vi "Get Time.vi"() -> (0 "time (ns)":u64)   [LabVIEW 2015, in "FPGA Timekeeper.lvlib"]
doc: "Returns the current time of the FPGA Timekeeper."
uses:
  FPGA Timekeeper.lvlib
  private/time (g).vi
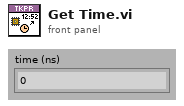
[diagram p1: front panel]
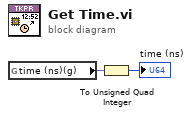
[diagram p0: block diagram]
diagram:
  n1 = global read "time (g).vi" "time (ns)(g)"() -> (w2:fxp<+,64,64>)
  n2 = To Unsigned Quad Integer(1:w2) -> (0:→"time (ns)":u64)
